vi "Insert Data by String Array.vi"(7 "data":string[](array[string]), 8 "error in (no error)":errorcluster, 9 "columns":string[](array[string]), 10 "table":string, 11 "ADODB in":refnum<class "ADODB.lvclass">) -> (0 "error out":errorcluster, 3 "ADODB out":refnum<class "ADODB.lvclass">)   [LabVIEW 2020, in "ADODB.lvlib" / "ADODB.lvclass"]
uses:
  ADODB.lvclass
  ADODB.lvclass/ADODB.ctl
  <vilib>/addons/database/Connection.llb/Conn Execute.vi
  <vilib>/addons/database/Recordset.llb/Rec Destroy - Connection.vi
  DBMS Specific/DBMS Specific.lvclass
  <vilib>/addons/database/NI_Database_API.lvlib
panel:
  # "This VI does not correct for \"Data\" string formatting. \nI.e., most DBMS require non-numeric \nvalues to have single quotes around them, 'value'"
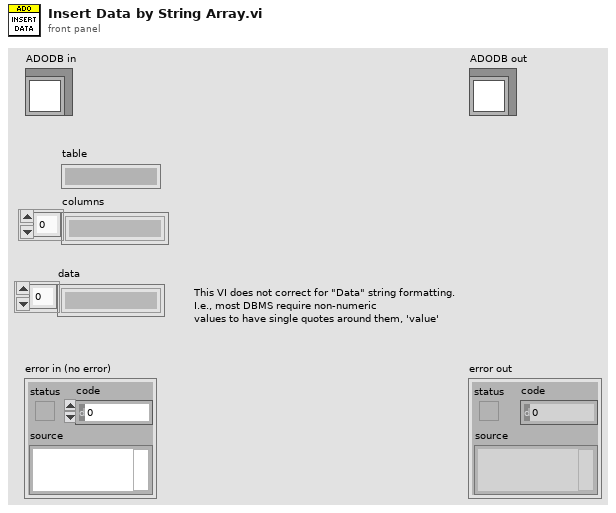
[diagram p1: front panel]
types:
  T1 = typedef "NI_Database_API.lvlib/Conn ObjectReference.ctl" = refnum<k1>
  T2 = typedef "NI_Database_API.lvlib/Rec ObjectReference.ctl" = refnum<k1>
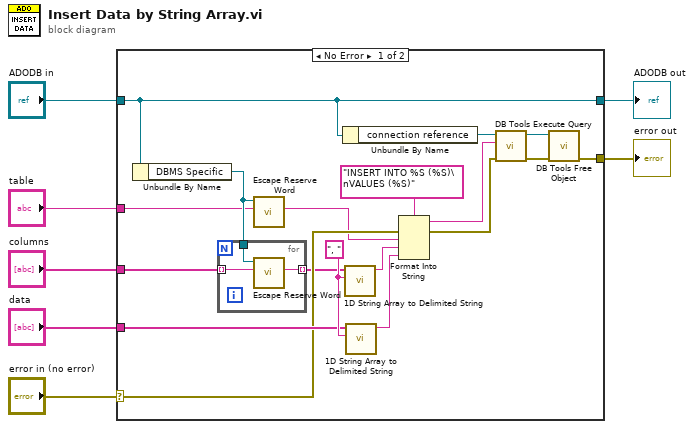
[diagram p0: block diagram]
diagram:
  n1 = case shown="No Error" "error in (no error)" {
    selector: "error in (no error)" -> [w15 w30]
    tunnel: "columns" -> [w9 _]
    tunnel: "data" -> [w23 _]
    tunnel: [w16 w30] -> w4
    tunnel: "ADODB in" -> [w12 w29]
    tunnel: [w12 w29] -> w2
    tunnel: "table" -> [w11 _]
    frame No Error {
      w24 = ", " ("delimiter")
      n2 = Unbundle By Name(w12) -> ("DBMS Specific"=w13:refnum<class "DBMS Specific.lvclass">)
      n3 = for {
        tunnel: w13 -> [w28]
        tunnel: w9 -> [w27] mode=indexing
        tunnel: [w26] -> w8 mode=indexing
        n4 = call-dynamic "Escape Reserve Word.vi"("Input Name"=w27, "DBMS Specific in"=w28) -> ("Escaped Name"=w26:string)  [unwired: 7 in, 2 out]
      }
      n5 = call-dynamic "Escape Reserve Word.vi"("Input Name"=w11, "DBMS Specific in"=w13) -> ("Escaped Name"=w10:string)  [unwired: 7 in, 2 out]
      n6 = Unbundle By Name(w12) -> ("connection reference"=w19:T1)
      n7 = call <vilib>:"1D String Array to Delimited String.vi"("delimiter"=w24, "string array"=w8) -> ("delimited string"=w22:string)  [unwired: 9 in]
      n8 = call <vilib>:"1D String Array to Delimited String.vi"("delimiter"=w24, "string array"=w23) -> ("delimited string"=w21:string)  [unwired: 9 in]
      n9 = Format Into String(format string="INSERT INTO %S (%S)\nVALUES (%S)", error in=w15, w10, w22, w21) -> (resulting string=w20:string, error out=w14:errorcluster)  [unwired: 1 in]
      n10 = call-poly <vilib>:"DB Tools Execute Query.vi"("error in (no error)"=w14, "SQL query"=w20, "connection reference"=w19) -> ("error out"=w17:errorcluster, "recordset reference"=w18:T2)  [unwired: 5 in]
      n11 = call-poly <vilib>:"DB Tools Free Object.vi"("error in (no error)"=w17, "recordset reference"=w18) -> ("error out"=w16:errorcluster)  [unwired: 8 in, 1 out]
    }
    frame Error {
    }
  }
  "error out" <- w4
  "ADODB out" <- w2
